vi "test Endpoint_Connected_Sends Connected Message.vi"(8 "error in (no error)":errorcluster, 11 "TestCase in":refnum<class "Test Notifying Nested Endpoint.lvclass">) -> (0 "error out":errorcluster, 3 "TestCase out":refnum<class "Test Notifying Nested Endpoint.lvclass">)   [LabVIEW 2020, in "Test Notifying Nested Endpoint.lvclass"]
uses:
  Test Notifying Nested Endpoint.lvclass
  <vilib>/addons/_JKI Toolkits/VI Tester/TestCase.llb/TestCase.lvclass
  <vilib>/ActorFramework/Message Queue/Message Queue.lvclass
  <vilib>/ActorFramework/Message Dequeuer/Message Dequeuer.lvclass
  Source/Nested Endpoint Caller/Nested Endpoint Caller Messages/Endpoint Connected Msg/Endpoint Connected Msg.lvclass
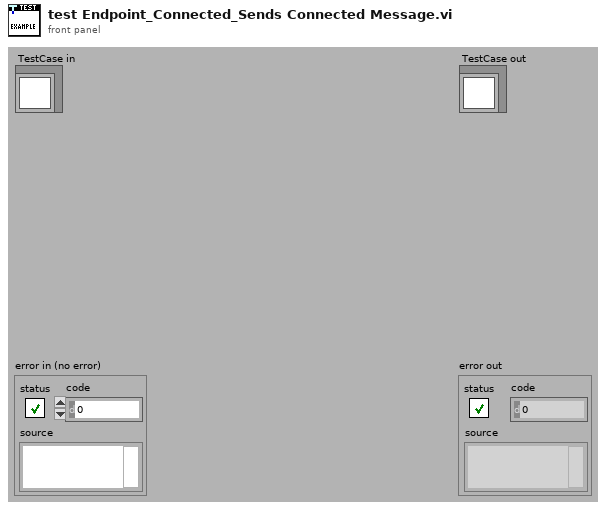
[diagram p1: front panel]
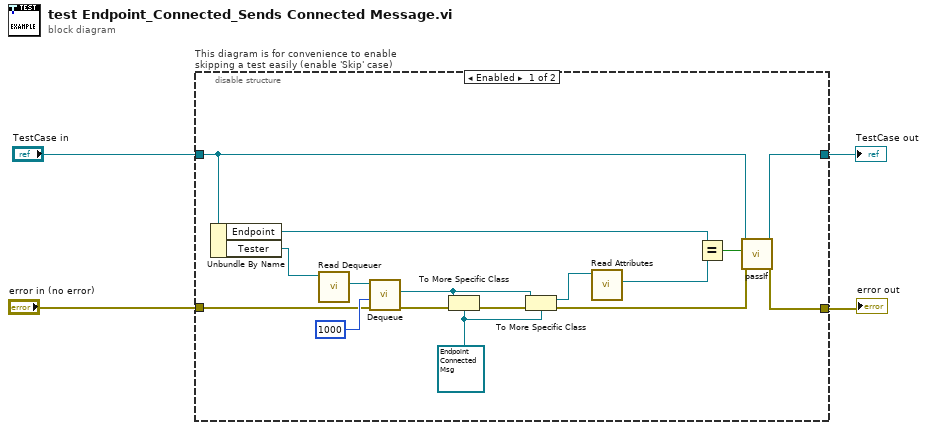
[diagram p0: block diagram]
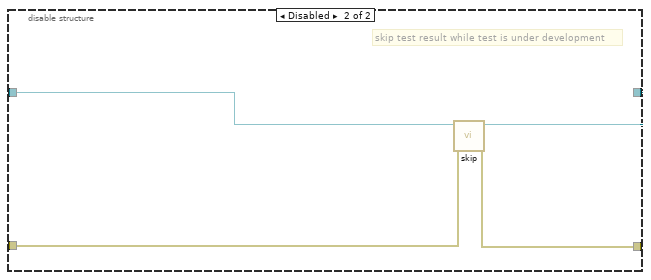
[diagram p2: hidden frame]
diagram:
  n1 = disable-structure "This diagram is for convenience to enable skipping a test easily (enable 'Skip' case)" shown="Enabled" {
    disable-tunnel: "TestCase in" -> [w18 w24]
    disable-tunnel: [w20 w22] -> w1
    disable-tunnel: [w19 w23] -> w3
    disable-tunnel: "error in (no error)" -> [w9 w21]
    frame Enabled {
      w6 = refnum<class "Endpoint Connected Msg.lvclass"> refnum ("Nested Endpoint Caller.lvlib:Endpoint Connected Msg.lvclass")
      n2 = Unbundle By Name(w18) -> ("Endpoint"=w7:refnum<class "Message Enqueuer.lvclass">, "Tester"=w17:refnum<class "Message Queue.lvclass">)
      n3 = call <vilib>:"Read Dequeuer.vi"("Message Queue"=w17) -> ("Message Dequeuer"=w16:refnum<class "Message Dequeuer.lvclass">)  [unwired: 10 in]
      n4 = call <vilib>:"Dequeue.vi"("error in (no error)"=w9, "timeout in ms (-1)"=1000, "Message Dequeuer in"=w16) -> ("error out"=w13:errorcluster, "Message"=w11:refnum<class "Message.lvclass">)  [unwired: 4 in, 3 out]
      n5 = To More Specific Class(target class=w6, reference=w11, error in=w13) -> (error out=w12:errorcluster)  [unwired: 1 out]
      n6 = To More Specific Class(target class=w6, reference=w11, error in=w12) -> (specific class reference=w10:refnum<class "Endpoint Connected Msg.lvclass">, error out=w8:errorcluster)
      n7 = call "Read Attributes.vi"("Endpoint Connected Msg in"=w10) -> ("Endpoint"=w5:refnum<class "Message Enqueuer.lvclass">)  [unwired: 10 in]
      n8 = Equal?(x=w7, y=w5) -> (x = y?=w15:bool)
      n9 = call-dynamic "passIf.vi"("error in (no error)"=w8, "pass"=w15, "TestCase in"=w18) -> ("error out"=w19:errorcluster, "TestCase out"=w20:refnum<class "Test Notifying Nested Endpoint.lvclass">)  [unwired: 7 in]
    }
    frame Disabled {
      # "skip test result while test is under development"
      n10 = call <vilib>:"skip.vi"("error in (no error)"=w21, "TestCase in"=w24) -> ("error out"=w23:errorcluster, "TestCase out"=w22:refnum<class "Test Notifying Nested Endpoint.lvclass">)  [unwired: 8 in]
    }
  }
  "error out" <- w3
  "TestCase out" <- w1
